vi "SetWavePt.vi"(9 "Voltage":sgl, 10 "DaNum":u8, 11 "error in":errorcluster caption="错误输入") -> (3 "error out":errorcluster caption="错误输出")   [LabVIEW 2016]
uses:
  PLC-Lab/lib/gusb.dll
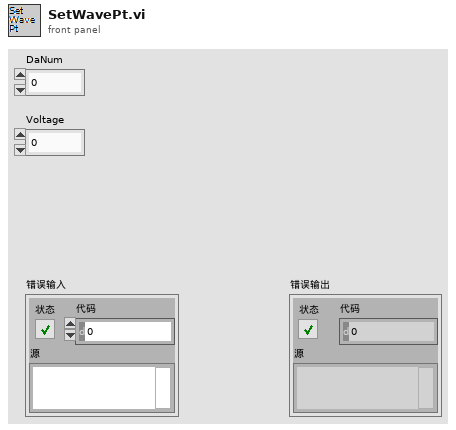
[diagram p1: front panel]
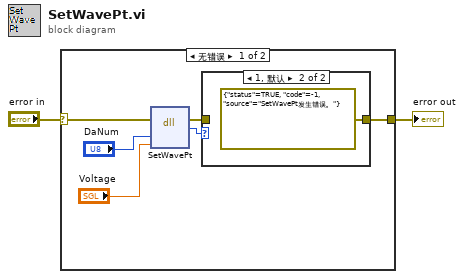
[diagram p0: block diagram]
diagram:
  n1 = case shown="无错误" "error in" {
    selector: "error in" -> [w8 w11]
    tunnel: [w6 w11] -> w1
    frame No Error {
      n2 = dll-call lib="E:/Camproject/2018/2018.1Labview/PLC-Lab/lib/gusb.dll" fn="SetWavePt"(error in=w8, "DANum"="DaNum", "Voltage"="Voltage") -> (error out=w5:errorcluster, "Status"=w7:i32)  [unwired: 4 in, 1 out]
      n3 = case shown="1, 默认" w7 {
        tunnel: w5 -> [w9 _]
        tunnel: [w9 errorcluster {"status"=TRUE, "code"=-1, "source"="SetWavePt发生错误。"} ("错误常量")] -> w6
        frame 0 {
        }
        frame 1, Default {
        }
      }
    }
    frame Error {
    }
  }
  "error out" <- w1
